vi "Init MCP.vi"(8 "error in (no error)":errorcluster, 11 "Data Cluster in":T1) -> (0 "error out":errorcluster, 3 "Data Cluster out":T1)   [LabVIEW 2025, in "Scripting Server.lvlib"]
uses:
  Scripting Server.lvlib
  Module Data--cluster.ctl
  Config Data.ctl
  open_vi.vi
  create_project.vi
  get_allowed_paths.vi
  get_structure_diagram.vi
  get_loop_iteration_terminal.vi
  show_conditional_terminal.vi
  get_loop_conditional_terminal.vi
  get_object_help.vi
  connect_to_pane.vi
  add_subvi.vi
  set_value.vi
  save_vi.vi
  delete_object.vi
  enclose_selection.vi
  rename_object.vi
  add_to_selection.vi
  remove_from_selection.vi
  clear_selection_list.vi
  run_vi.vi
  create_control.vi
  cleanup_vi.vi
  get_vi_error_list.vi
  get_object_terminals.vi
  connect_objects.vi
  new_vi.vi
  add_object.vi
  get_library.vi
  get_vi_blockdiagram.vi
  Get VI Frontpanel Picture.vi
  <vilib>/jgoebel/LabVIEW MCP Server SDK/MCP Server.lvlib
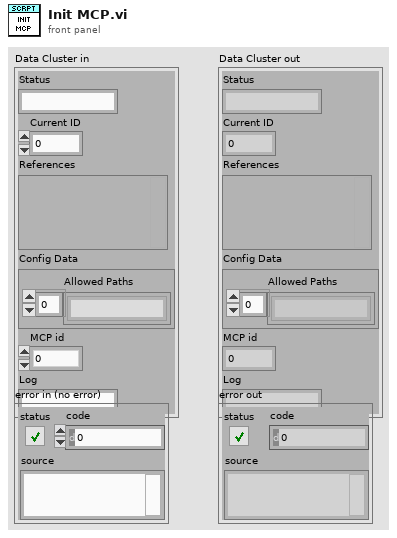
[diagram p1: front panel]
types:
  T1 = typedef "Scripting Server.lvlib/Module Data--cluster.ctl" = cluster{"Status":string, "Current ID":i32, "References":variant, "Config Data":T2, "MCP id":i32, "Log":string}
  T2 = typedef "Scripting Server.lvlib/Config Data.ctl" = cluster{"Allowed Paths":string[]}
  T3 = typedef "MCP Server.lvlib/User Events.ctl" = cluster{"onError":refnum<user-event>, "onRpc":refnum<user-event>}
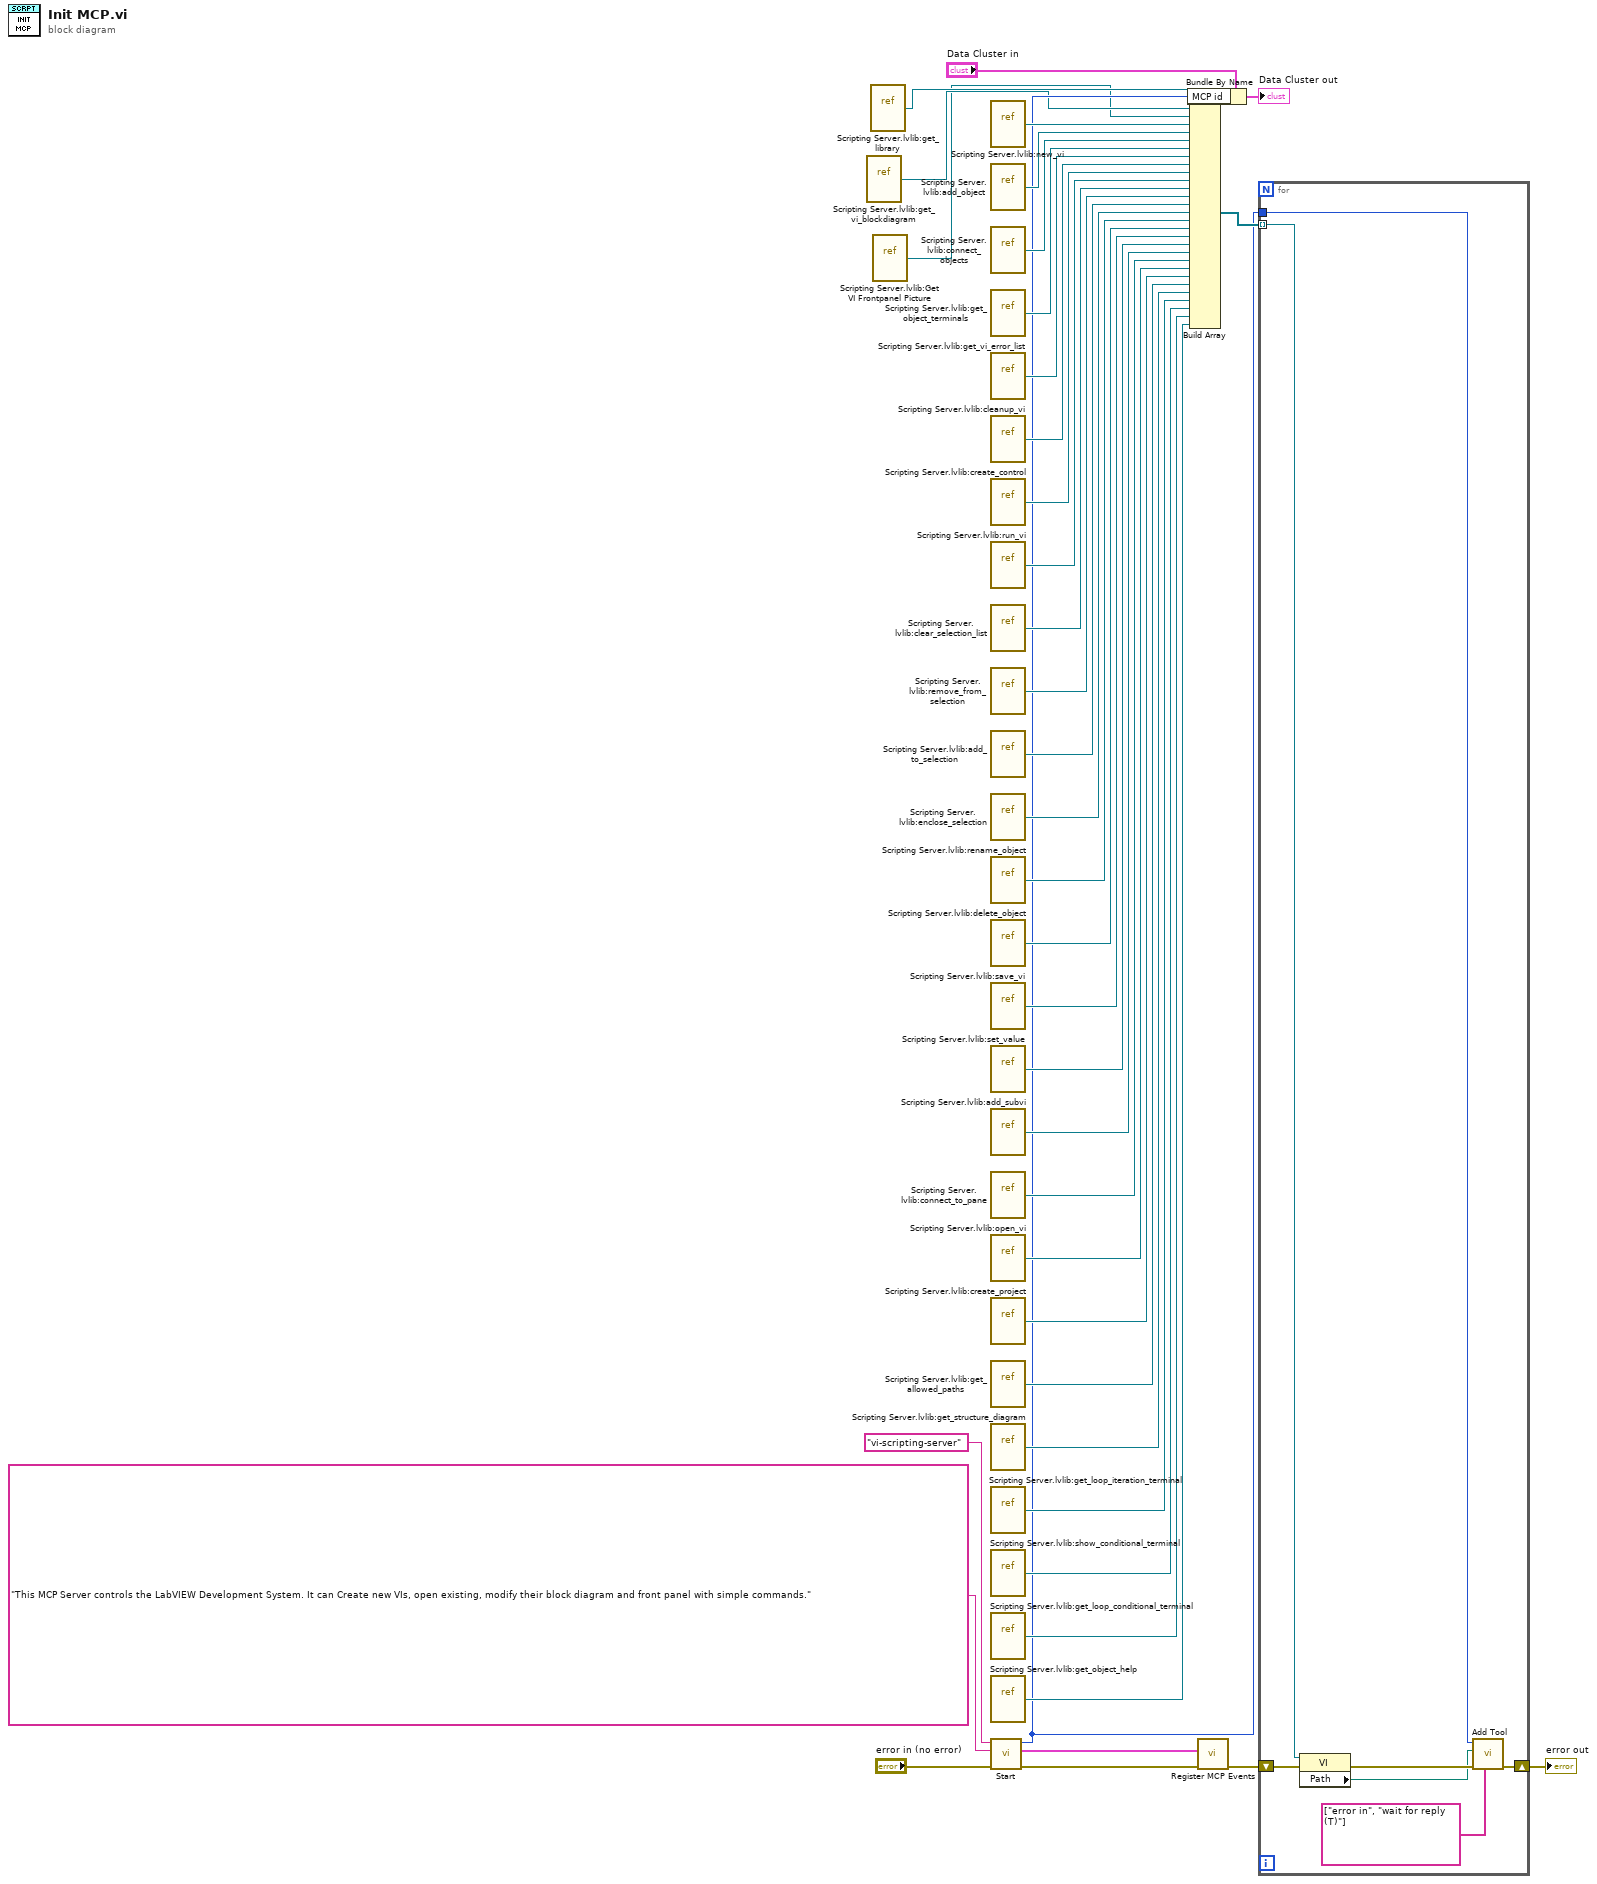
[diagram p0: block diagram]
diagram:
  n1 = vi-ref "Scripting Server.lvlib:get_vi_blockdiagram.vi"() -> (w2:refnum<vi>)
  n2 = vi-ref "Scripting Server.lvlib:get_library.vi"() -> (w3:refnum<vi>)
  n3 = vi-ref "Scripting Server.lvlib:Get VI Frontpanel Picture.vi"() -> (w1:refnum<vi>)
  n4 = vi-ref "Scripting Server.lvlib:new_vi.vi"() -> (w36:refnum<vi>)
  n5 = vi-ref "Scripting Server.lvlib:add_object.vi"() -> (w35:refnum<vi>)
  n6 = vi-ref "Scripting Server.lvlib:connect_objects.vi"() -> (w34:refnum<vi>)
  n7 = vi-ref "Scripting Server.lvlib:get_object_terminals.vi"() -> (w33:refnum<vi>)
  n8 = vi-ref "Scripting Server.lvlib:get_vi_error_list.vi"() -> (w32:refnum<vi>)
  n9 = vi-ref "Scripting Server.lvlib:cleanup_vi.vi"() -> (w31:refnum<vi>)
  n10 = vi-ref "Scripting Server.lvlib:create_control.vi"() -> (w30:refnum<vi>)
  n11 = vi-ref "Scripting Server.lvlib:run_vi.vi"() -> (w29:refnum<vi>)
  n12 = vi-ref "Scripting Server.lvlib:clear_selection_list.vi"() -> (w28:refnum<vi>)
  n13 = vi-ref "Scripting Server.lvlib:remove_from_selection.vi"() -> (w27:refnum<vi>)
  n14 = vi-ref "Scripting Server.lvlib:add_to_selection.vi"() -> (w26:refnum<vi>)
  n15 = vi-ref "Scripting Server.lvlib:enclose_selection.vi"() -> (w24:refnum<vi>)
  n16 = vi-ref "Scripting Server.lvlib:rename_object.vi"() -> (w25:refnum<vi>)
  n17 = vi-ref "Scripting Server.lvlib:delete_object.vi"() -> (w23:refnum<vi>)
  n18 = vi-ref "Scripting Server.lvlib:save_vi.vi"() -> (w22:refnum<vi>)
  n19 = vi-ref "Scripting Server.lvlib:set_value.vi"() -> (w21:refnum<vi>)
  n20 = vi-ref "Scripting Server.lvlib:add_subvi.vi"() -> (w20:refnum<vi>)
  n21 = vi-ref "Scripting Server.lvlib:connect_to_pane.vi"() -> (w19:refnum<vi>)
  n22 = vi-ref "Scripting Server.lvlib:open_vi.vi"() -> (w18:refnum<vi>)
  n23 = vi-ref "Scripting Server.lvlib:create_project.vi"() -> (w17:refnum<vi>)
  n24 = vi-ref "Scripting Server.lvlib:get_allowed_paths.vi"() -> (w16:refnum<vi>)
  n25 = vi-ref "Scripting Server.lvlib:get_structure_diagram.vi"() -> (w15:refnum<vi>)
  n26 = vi-ref "Scripting Server.lvlib:get_loop_iteration_terminal.vi"() -> (w14:refnum<vi>)
  n27 = vi-ref "Scripting Server.lvlib:show_conditional_terminal.vi"() -> (w13:refnum<vi>)
  n28 = vi-ref "Scripting Server.lvlib:get_loop_conditional_terminal.vi"() -> (w12:refnum<vi>)
  n29 = vi-ref "Scripting Server.lvlib:get_object_help.vi"() -> (w11:refnum<vi>)
  n30 = call <vilib>:"Start.vi"("error in (no error)"="error in (no error)", "Description"="This MCP Server controls the LabVIEW Development System. It can Create new VIs, open existing, modify their block diagram and front panel with simple commands.", "Name"="vi-scripting-server") -> ("error out"=w7:errorcluster, "MCP Events"=w6:T3, "server id out"=w5:i32)  [unwired: 6 in]
  n31 = Bundle By Name(cluster="Data Cluster in", "MCP id"=w5) -> (→"Data Cluster out":T1)
  n32 = Build Array(w3, w2, w1, w36, w35, w34, w33, w32, w31, w30, w29, w28, w27, w26, w24, w25, w23, w22, w21, w20, w19, w18, w17, w16, w15, w14, w13, w12, w11) -> (w10:refnum<vi>[])
  n33 = call "Register MCP Events.vi"("error in"=w7, "MCP Events"=w6) -> ("error out"=w38:errorcluster)  [unwired: 9 in]
  n34 = for {
    shift-right: [w43] -> w37
    shift-left: w38 -> [w47]
    tunnel: w10 -> [w46] mode=indexing
    tunnel: w5 -> [w45]
    n35 = property class="VI"(reference=w46, error in=w47) -> (error out=w44:errorcluster, "Path"=w42:path)  [unwired: 1 out]
    n36 = call <vilib>:"Add Tool.vi"("Ignored"=string[] ["error in", "wait for reply (T)"], "error in (no error)"=w44, "vi path"=w42, "server id"=w45) -> ("error out"=w43:errorcluster)  [unwired: 6 in, 1 out]
  }
  "error out" <- w37
